vi "PH_Tektronix_7000.convert Bandwidth.vi"(1 "Bandwidth raw":string) -> (0 "Bandwidth":u16(ring) items=["FULL", "500 MHz", "250 MHz", "150 MHz", "20 MHz"])   [LabVIEW 2014, in "PH_Tektronix_7000.lvlib"]
doc: "This VI calculates from the raw bandwidth (string) a possible bandwidth (to be 20MHz, 150MHz, 250MHz, 500MHz, or FULL (which is default)."
uses:
  PH_Tektronix_7000.lvlib
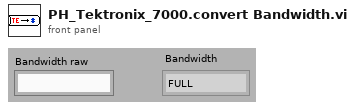
[diagram p1: front panel]
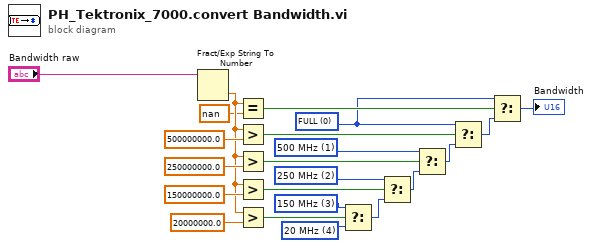
[diagram p0: block diagram]
diagram:
  w6 = u16 4 items=["FULL", "500 MHz", "250 MHz", "150 MHz", "20 MHz"] ("Bandwidth")
  w9 = u16 3 items=["FULL", "500 MHz", "250 MHz", "150 MHz", "20 MHz"] ("Bandwidth")
  w12 = u16 2 items=["FULL", "500 MHz", "250 MHz", "150 MHz", "20 MHz"] ("Bandwidth")
  w16 = u16 1 items=["FULL", "500 MHz", "250 MHz", "150 MHz", "20 MHz"] ("Bandwidth")
  w2 = u16 0 items=["FULL", "500 MHz", "250 MHz", "150 MHz", "20 MHz"] ("Bandwidth")
  n1 = Fract/Exp String To Number(string="Bandwidth raw") -> (number=w5:dbl)  [unwired: 3 in, 1 out]
  n2 = Equal?(x=w5, y=nan) -> (x = y?=w3:bool)
  n3 = Greater?(x=w5, y=500000000.0) -> (0:w19:bool)
  n4 = Greater?(x=w5, y=250000000.0) -> (0:w17:bool)
  n5 = Greater?(x=w5, y=150000000.0) -> (0:w11:bool)
  n6 = Greater?(x=w5, y=20000000.0) -> (0:w7:bool)
  n7 = Select(t=w9, s=w7, f=w6) -> (s? t:f=w8:u16)
  n8 = Select(t=w12, s=w11, f=w8) -> (s? t:f=w10:u16)
  n9 = Select(t=w16, s=w17, f=w10) -> (s? t:f=w15:u16)
  n10 = Select(t=w2, s=w19, f=w15) -> (s? t:f=w1:u16)
  n11 = Select(t=w2, s=w3, f=w1) -> (s? t:f=→"Bandwidth":u16)
